vi "Wait_for_Equilibrium.vi"(0 "error in":errorcluster) -> (2 "error out":errorcluster, 3 "Difference":dbl, 4 "Temperature Error":dbl, 5 "Temperature Mean":dbl)   [LabVIEW 2010]
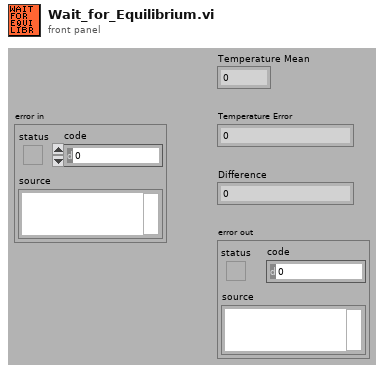
[diagram p1: front panel]
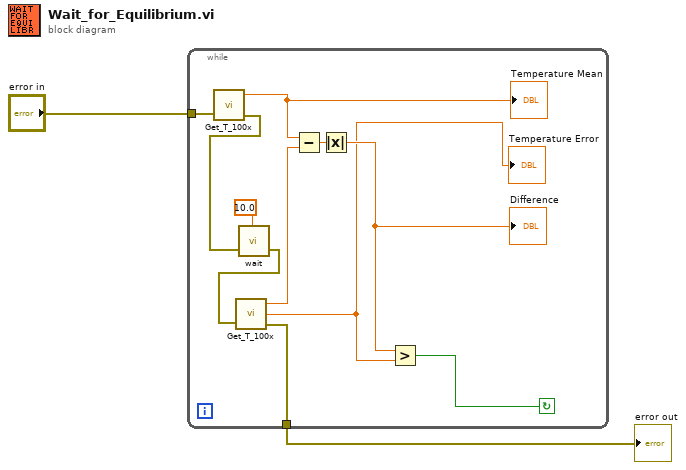
[diagram p0: block diagram]
diagram:
  n1 = while {
    tunnel: "error in" -> [w10]
    tunnel: [w5] -> w1
    stop <- w11 continue-if-true
    n2 = call "Get_T_100x.vi"("error in"=w10) -> ("error out"=w12:errorcluster, "Temperature Mean"=w8:dbl)  [unwired: 1 in, 1 out]
    "Temperature Mean" <- w8
    n3 = call "wait.vi"("error in"=w12, "Wartezeit in Sek"=10.0) -> ("error out"=w6:errorcluster)  [unwired: 1 in]
    n4 = call "Get_T_100x.vi"("error in"=w6) -> ("error out"=w5:errorcluster, "Temperature Error"=w3:dbl, "Temperature Mean"=w4:dbl)  [unwired: 1 in]
    "Temperature Error" <- w3
    n5 = Subtract(x=w8, y=w4) -> (x-y=w13:dbl)
    n6 = Absolute Value(x=w13) -> (abs(x)=w7:dbl)
    "Difference" <- w7
    n7 = Greater?(x=w7, y=w3) -> (0:w11:bool)
  }
  "error out" <- w1
